vi "Set Column Type.vi"(8 "error in (no error)":errorcluster, 10 "Column Type":T1, 11 "Column Configuration in":refnum<class "Column Configuration.lvclass">) -> (0 "error out":errorcluster, 3 "Column Configuration out":refnum<class "Column Configuration.lvclass">)   [LabVIEW 2020, in "Column Interfaces.lvlib" / "Column Configuration.lvclass"]
uses:
  Column Configuration.lvclass
  Database Libraries/Database Interfaces/Database data type.ctl
  Database Libraries/Database Interfaces.lvlib
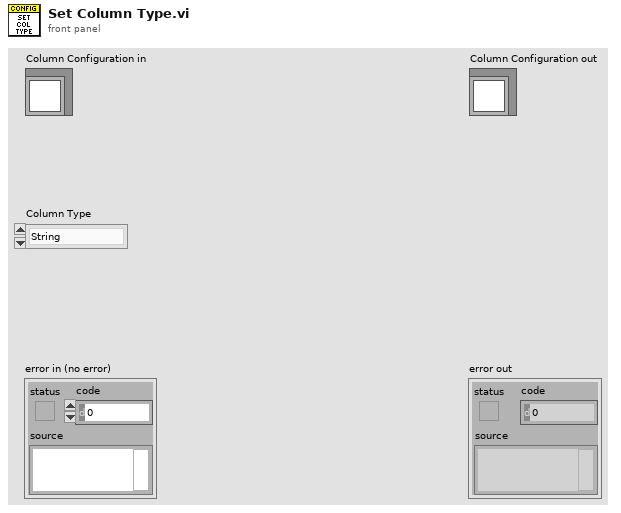
[diagram p1: front panel]
types:
  T1 = typedef "Database Interfaces.lvlib/Database data type.ctl" = enum16{"String", "Long (I32)", "Single (SGL)", "Double (DBL)", "Date/Time", "Binary"}
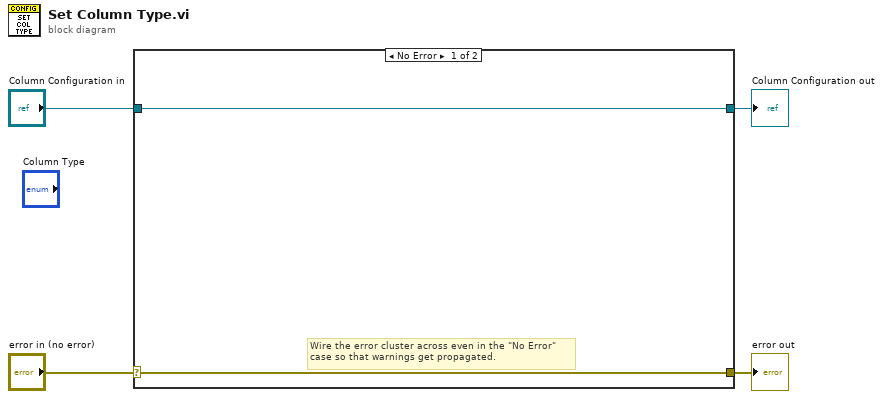
[diagram p0: block diagram]
diagram:
  n1 = case shown="No Error" "error in (no error)" {
    selector: "error in (no error)" -> [w5 w8]
    tunnel: [w5 w8] -> w3
    tunnel: [w6 w7] -> w1
    tunnel: "Column Configuration in" -> [w6 w7]
    frame No Error {
      # "Wire the error cluster across even in the \"No Error\"\ncase so that warnings get propagated."
    }
    frame Error {
    }
  }
  "error out" <- w3
  "Column Configuration out" <- w1
